vi "Detect Target - Auto Threshold.vi"(0 "Image":T1, 1 "Image Mask":T1, 2 "Image Buffer":T1) -> (3 "Original Image":T1(plugin-control), 4 "X":i16, 5 "Y":i16, 6 "Found Target":bool)   [LabVIEW 2015]
uses:
  Camera Types.ctl
  <vilib>/vision/Image Controls.llb/IMAQ Image.ctl
  <vilib>/vision/NI_Vision_Development_Module.lvlib
panel:
  out "Threshold Data out":T2(array[cluster]) {"Replace Value" format="%.2f"; "Upper value" format="%.2f"; "Lower value" format="%.2f"}
  in  "Number of Classes":i32=4
  out "Detected Targets":T3(array[cluster]) {"Normalized Rect"."Numeric 5" format="%#_2g"; "Normalized Rect"."Numeric 3" format="%#_2g"; "Normalized Rect"."Numeric 2" format="%#_2g"; "Normalized Rect"."Numeric" format="%#_2g"}
  out "Highest Avg Score":dbl
  out "Sorted Particle Scores":T4(array[cluster]) {"Moment Factor" format="%#_3g"; "Aspect Ratio" format="%#_3g"; "Area to CH" format="%#_3g"; "X" format="%#_3g"; "Y" format="%#_3g"}
  in  "Display Mask":bool=TRUE
  out "Masked":T1(plugin-control)
  in  "Emphasize Limit Tests":bool=TRUE
  in  "Camera Type":T5=enum."MS HD3000 square"
  in  "Min Score Threshold":i32=75
  in  "Aspect Fudge Factor":dbl=1.0
  out "Qualified Particles":i32
  # "Density Profile"
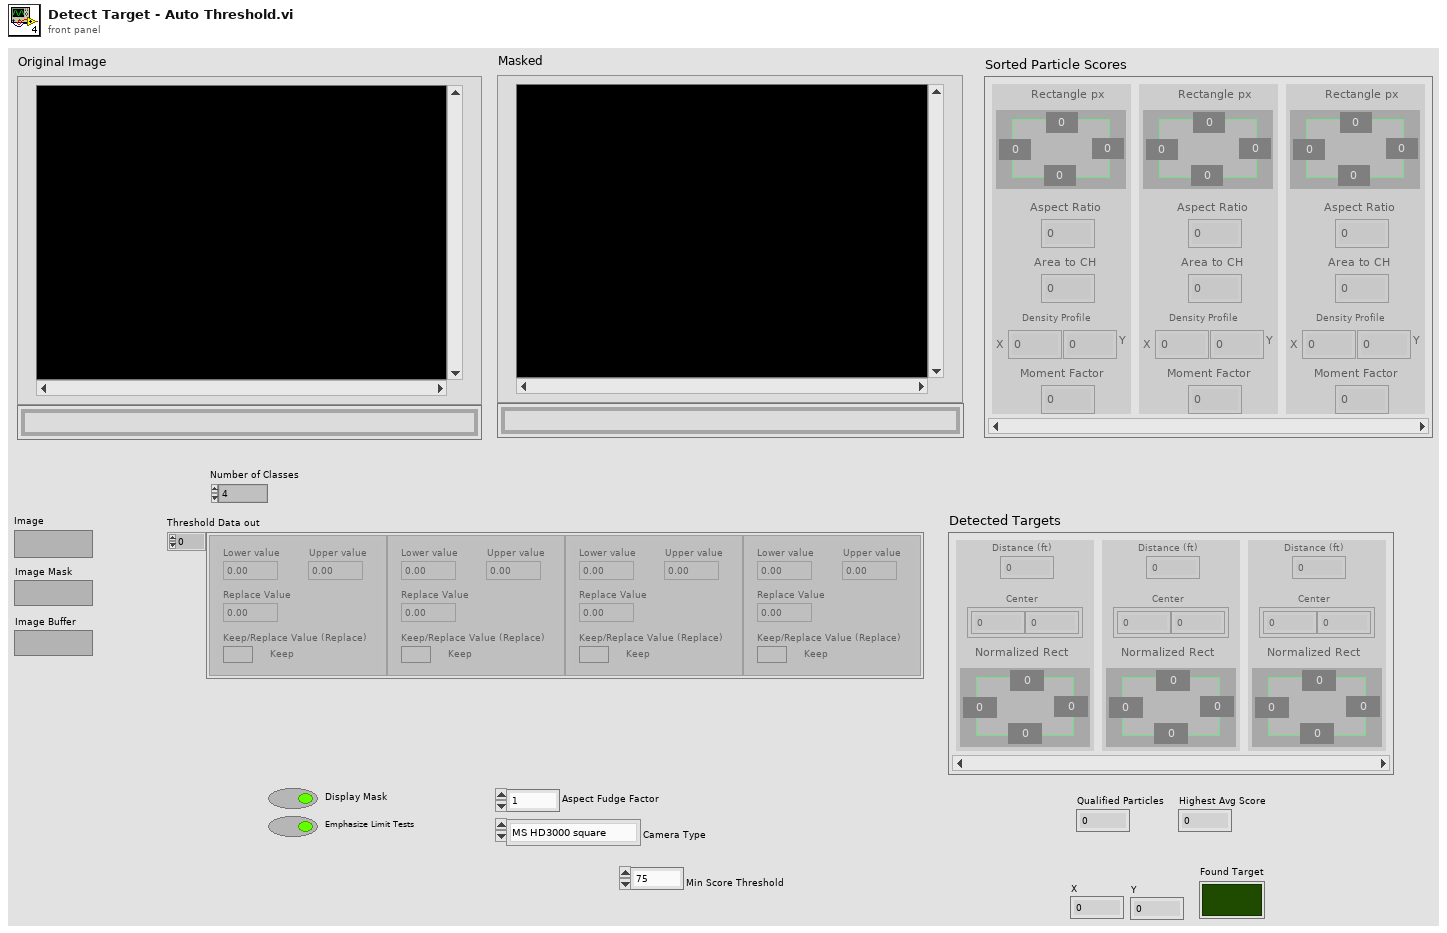
[diagram p1: front panel]
types:
  T1 = typedef "IMAQ Image.ctl" = refnum<image>
  T2 = cluster{"Lower value":sgl, "Upper value":sgl, "Replace Value":sgl, "Keep/Replace Value (Replace)":bool}[]
  T3 = cluster{"Distance (ft)":dbl, "Center":cluster{dbl, dbl}, "Normalized Rect":cluster{"Numeric":dbl, "Numeric 2":dbl, "Numeric 3":dbl, "Numeric 5":dbl}}[]
  T4 = cluster{"Rectangle px":cluster{"Numeric":dbl, "Numeric 2":dbl, "Numeric 3":dbl, "Numeric 5":dbl}, "Aspect Ratio":dbl, "Area to CH":dbl, "X":dbl, "Y":dbl, "Moment Factor":dbl}[]
  T5 = typedef "Camera Types.ctl" = enum16{"206", "1011", "1013", "MS HD3000 square", "MS HD3000 640x480"}
  T6 = typedef "Particle Parameters" = i32
  T7 = cluster{"Replace Value":sgl, "Replace Value":sgl}
  T8 = cluster{"Bounding box":cluster{"left":dbl, "top":dbl, "right":dbl, "bottom":dbl}, "Aspect Ratio":dbl, "Area to CH":dbl, "X Mask":dbl, "Y Mask":dbl, "Moment":dbl}[]
  T9 = cluster{"Rectangle":cluster{"Numeric":dbl, "Numeric 2":dbl, "Numeric 3":dbl, "Numeric 5":dbl}, "L":dbl, "Area to CH":dbl, "X":dbl, "Y":dbl, "Moment Factor":dbl}[]
  T10 = cluster{"Rectangle":cluster{"Numeric":dbl, "Numeric 2":dbl, "Numeric 3":dbl, "Numeric 5":dbl}, "L":dbl, "Area to CH":dbl, "X":dbl, "Y":dbl, "Moment Factor":dbl}
  T11 = cluster{"Numeric":dbl, "Numeric 2":dbl, "Numeric 3":dbl, "Numeric 5":dbl}
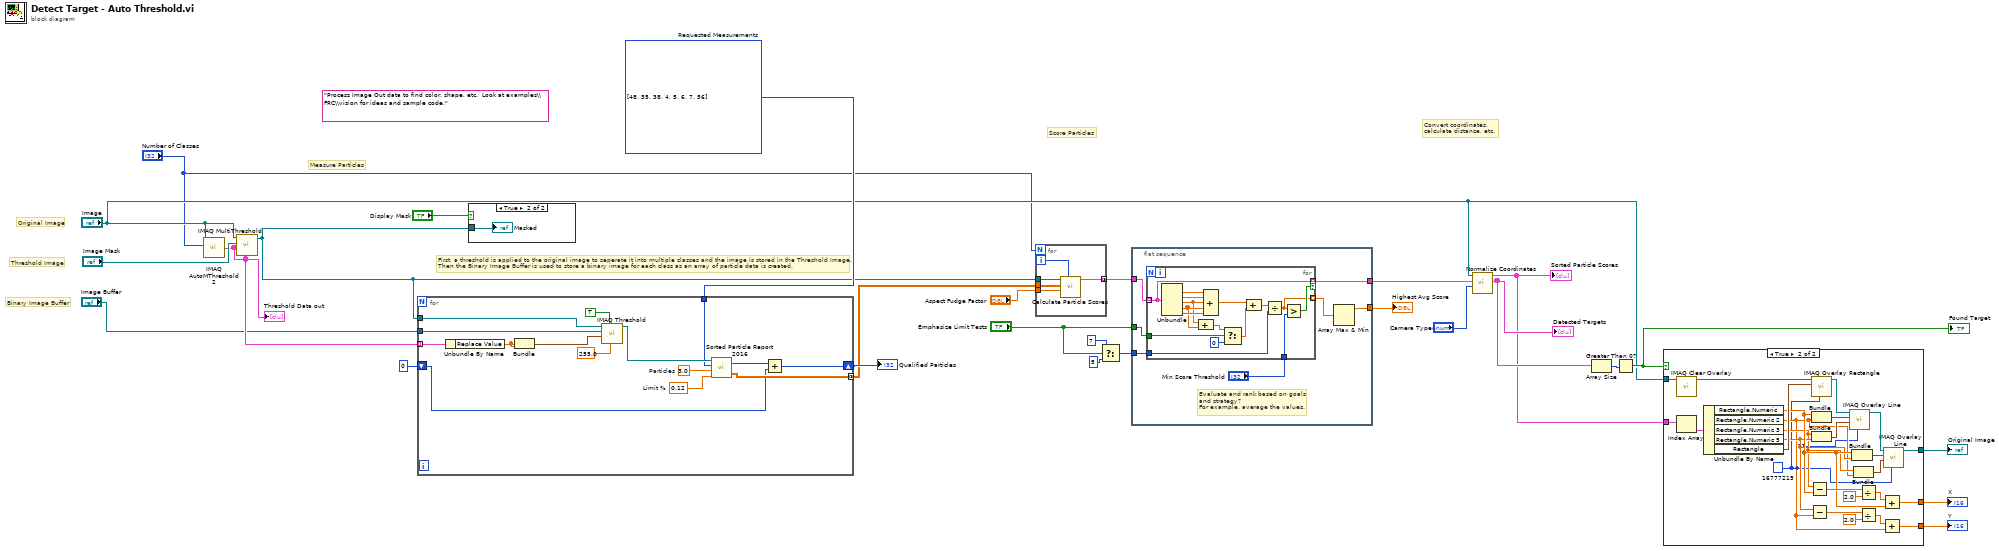
[diagram p0: block diagram]
diagram:
  w12 = T6[] [48, 35, 38, 4, 5, 6, 7, 56] items=["Center of Mass X", "Center of Mass Y", "First Pixel X", "First Pixel Y", "Bounding Rect Left", "Bounding Rect Top", "Bounding Rect Right", "Bounding Rect Bottom", "Max Feret Diameter Start X", "Max Feret Diameter Start Y", "Max Feret Diameter End X", "Max Feret Diameter End Y", "Max Horiz. Segment Length Left", "Max Horiz. Segment Length Right", "Max Horiz. Segment Length Row", "-", "Bounding Rect Width", "Bounding Rect Height", "Bounding Rect Diagonal", "Perimeter", "Convex Hull Perimeter", "Holes' Perimeter", "Max Feret Diameter", "Equivalent Ellipse Major Axis", "Equivalent Ellipse Minor Axis", "Equivalent Ellipse Minor Axis (Feret)", "Equivalent Rect Long Side", "Equivalent Rect Short Side", "Equivalent Rect Diagonal", "Equivalent Rect Short Side (Feret)", "Average Horiz. Segment Length", "Average Vert. Segment Length", "Hydraulic Radius", "Waddel Disk Diameter", "-", "Area", "Holes' Area", "Particle & Holes' Area", "Convex Hull Area", "Image Area", "-", "Number of Holes", "Number of Horiz. Segments", "Number of Vert. Segments", "-", "Orientation", "Max Feret Diameter Orientation", "-", "% Area/Image Area", "% Area/(Particle & Holes' Area)", "Ratio of Equivalent Ellipse Axes", "Ratio of Equivalent Rect Sides", "-", "Elongation Factor", "Compactness Factor", "Heywood Circularity Factor", "Type Factor", "-", "Sum X", "Sum Y", "Sum XX", "Sum XY", "Sum YY", "Sum XXX", "Sum XXY", "Sum XYY", "Sum YYY", "-", "Moment of Inertia XX", "Moment of Inertia XY", "Moment of Inertia YY", "Moment of Inertia XXX", "Moment of Inertia XXY", "Moment of Inertia XYY", "Moment of Inertia YYY", "Norm. Moment of Inertia XX", "Norm. Moment of Inertia XY", "Norm. Moment of Inertia YY", "Norm. Moment of Inertia XXX", "Norm. Moment of Inertia XXY", "Norm. Moment of Inertia XYY", "Norm. Moment of Inertia YYY", "Hu Moment 1", "Hu Moment 2", "Hu Moment 3", "Hu Moment 4", "Hu Moment 5", "Hu Moment 6", "Hu Moment 7"]  # Requested Measurements
  (unwired) "Process Image Out data to find color, shape, etc.  Look at examples\\FRC\\vision for ideas and sample code."
  # "First, a threshold is applied to the original image to seperate it into multiple classes and the image is stored in the Threshold Image.\nThen the Binary Image Buffer is used to store a binary image for each class as an array of particle data is created."
  # "Original Image"
  # "Threshold Image"
  # "Binary Image Buffer"
  # "Measure Particles"
  # "Convert coordinates,\ncalculate distance, etc."
  # "Score Particles"
  n1 = call "IMAQ AutoMThreshold 2"("Number of Classes"="Number of Classes", "Image"="Image") -> ("Threshold Data out"=w15:T2)  [unwired: 2 in, 2 out]
  "Threshold Data out" <- w15
  n2 = call "IMAQ MultiThreshold"("Threshold Data"=w15, "Image Dst"="Image Mask", "Image Src"="Image") -> ("Image Dst Out"=w1:T1)  [unwired: 2 in, 1 out]
  n3 = for {
    tunnel: w15 -> [w41] mode=indexing
    tunnel: "Image Buffer" -> [w40]
    tunnel: w1 -> [w39]
    tunnel: w12 -> [w33]
    tunnel: [w32] -> w13 mode=concatenating
    shift-right: [w31] -> w14
    shift-left: 0 -> [w30]
    w36 = 0.12  # Limit %
    w35 = 3.0  # Particles
    n4 = Unbundle By Name(w41) -> ("Replace Value"=w28:sgl)
    n5 = Bundle("Replace Value"=w28, "Replace Value"=w28) -> (w42:T7)  [unwired: 1 in]
    n6 = call "IMAQ Threshold"("Replace Value"=sgl 255.0, "Keep/Replace Value (Replace)"=TRUE, "Range"=w42, "Image Dst"=w40, "Image Src"=w39) -> ("Image Dst Out"=w34:T1)  [unwired: 5 in, 1 out]
    n7 = call "Sorted Particle Report 2016.vi"("Min Area Size %"=w36, "Particle Count Limit"=w35, "Pixel Measurements"=w33, "Image in"=w34) -> ("Sorted Data"=w32:dbl[][], "Particles"=w29:i32)
    n8 = Add(x=w29, y=w30) -> (x+y=w31:i32)
  }
  "Qualified Particles" <- w14
  n9 = case shown="True" "Display Mask" {
    tunnel: w1 -> [_ w43]
    frame False {
    }
    frame True {
      "Masked" <- w43
    }
  }
  n10 = for {
    N: "Number of Classes" -> [_]
    tunnel: "Aspect Fudge Factor" -> [w48]
    tunnel: [w47] -> w25 mode=concatenating
    tunnel: w1 -> [w46]
    tunnel: w13 -> [w45]
    i -> [w44]
    n11 = call "Calculate Particle Scores.vi"("Pixel Value"=w44, "Aspect Fudge Factor"=w48, "Sorted Data"=w45, "Image in"=w46) -> ("Scores"=w47:T8)  [unwired: 7 in]
  }
  n12 = Select(t=7, s="Emphasize Limit Tests", f=5) -> (s? t:f=w22:i32)
  n13 = flat-sequence {
    tunnel: w25 -> [w54]
    tunnel: w22 -> [w52]
    tunnel: [w55] -> w21
    tunnel: [w49] -> w19
    tunnel: "Emphasize Limit Tests" -> [w53]
    frame #0 {
      # "Evaluate and rank based on goals\nand strategy?\nFor example, average the values."
      n14 = for {
        tunnel: w54 -> [w69] mode=indexing
        tunnel: [w69] -> w49 mode=indexing if=w68
        tunnel: [w67] -> w50 mode=indexing
        tunnel: w52 -> [w66]
        tunnel: "Min Score Threshold" -> [w65]
        tunnel: w53 -> [w58]
        n15 = Unbundle(w69) -> ("Aspect Ratio"=w71:dbl, "Area to CH"=w70:dbl, "X Mask"=w60:dbl, "Y Mask"=w61:dbl, "Moment"=w62:dbl)  [unwired: 1 out]
        n16 = Compound Arithmetic op=ADD(w60, w61) -> (w59:dbl)
        n17 = Compound Arithmetic op=ADD(w71, w70, w60, w61, w62) -> (w64:dbl)
        n18 = Select(t=w59, s=w58, f=0) -> (s? t:f=w57:dbl)
        n19 = Compound Arithmetic op=ADD(w64, w57) -> (w63:dbl)
        n20 = Divide(x=w63, y=w66) -> (x/y=w67:dbl)
        n21 = Greater?(x=w67, y=w65) -> (0:w68:bool)
      }
      n22 = Array Max & Min(array=w50) -> (max value=w55:dbl)  [unwired: 3 out]
    }
  }
  n23 = call "Normalize Coordinates.vi"("Camera Type"="Camera Type", "Targets"=w19, "Image in"="Image") -> ("Found Targets"=w8:T3, "Sorted Scores"=w7:T9)  [unwired: 7 in]
  "Sorted Particle Scores" <- w7
  "Detected Targets" <- w8
  n24 = Array Size(array=w8) -> (size(s)=w10:i32)
  n25 = Greater Than 0?(x=w10) -> (x > 0?=w9:bool)
  "Found Target" <- w9
  n26 = case shown="True" w9 {
    tunnel: w7 -> [_ w97]
    tunnel: [_ w92] -> w4
    tunnel: [_ w88] -> w3
    tunnel: "Image" -> [w72 w85]
    tunnel: [w72 w80] -> w2
    frame False {
    }
    frame True {
      w73 = u32 16777215 ("Color")
      n27 = call "IMAQ Clear Overlay"("Image"=w85) -> ("Image Out"=w86:T1)  [unwired: 2 in, 8 out]
      n28 = Index Array(array=w97) -> (element=w96:T10)  [unwired: 1 in]
      n29 = Unbundle By Name(w96) -> ("Rectangle.Numeric"=w77:dbl, "Rectangle.Numeric 2"=w74:dbl, "Rectangle.Numeric 3"=w75:dbl, "Rectangle.Numeric 5"=w76:dbl, "Rectangle"=w87:T11)
      n30 = Subtract(x=w75, y=w77) -> (x-y=w94:dbl)
      n31 = Subtract(x=w76, y=w74) -> (x-y=w90:dbl)
      n32 = call "IMAQ Overlay Rectangle"("Color"=w73, "Rectangle"=w87, "Image"=w86) -> ("Image Out"=w84:T1)  [unwired: 7 in, 1 out]
      n33 = Bundle("Numeric"=w77, "Numeric 2"=w74) -> (w83:cluster{"Numeric":dbl, "Numeric 2":dbl})  [unwired: 1 in]
      n34 = Bundle("Numeric 3"=w75, "Numeric 5"=w76) -> (w82:cluster{"Numeric 3":dbl, "Numeric 5":dbl})  [unwired: 1 in]
      n35 = call "IMAQ Overlay Line"("Color"=w73, "End Point"=w82, "Start Point"=w83, "Image"=w84) -> ("Image Out"=w81:T1)  [unwired: 6 in, 1 out]
      n36 = Bundle("Numeric"=w77, "Numeric 5"=w76) -> (w79:cluster{"Numeric":dbl, "Numeric 5":dbl})  [unwired: 1 in]
      n37 = Bundle("Numeric 3"=w75, "Numeric 2"=w74) -> (w78:cluster{"Numeric 3":dbl, "Numeric 2":dbl})  [unwired: 1 in]
      n38 = Divide(x=w94, y=2.0) -> (x/y=w93:dbl)
      n39 = Divide(x=w90, y=2.0) -> (x/y=w89:dbl)
      n40 = Add(x=w93, y=w77) -> (x+y=w92:dbl)
      n41 = Add(x=w89, y=w74) -> (x+y=w88:dbl)
      n42 = call "IMAQ Overlay Line"("Color"=w73, "End Point"=w78, "Start Point"=w79, "Image"=w81) -> ("Image Out"=w80:T1)  [unwired: 6 in, 1 out]
    }
  }
  "X" <- w4
  "Y" <- w3
  "Original Image" <- w2
  "Highest Avg Score" <- w21
